vi "control_enabled_state.vi"(8 "error in (no error)":errorcluster, 10 "enabled":bool, 11 "control in":refnum<vi>) -> (0 "error out":errorcluster, 1 "disabled":bool, 2 "enabled":bool, 3 "control out":refnum<vi>)   [LabVIEW 2013, in "dsdll.lvlib"]
doc: "Enables or disables and grays references control."
uses:
  dsdll.lvlib
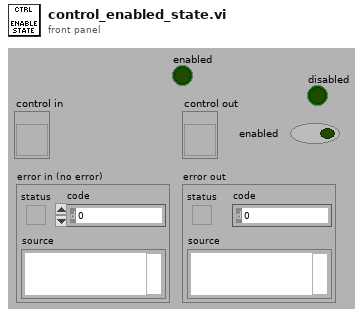
[diagram p1: front panel]
types:
  T1 = enum8{"Enabled", "Disabled", "Disabled and Grayed Out"}
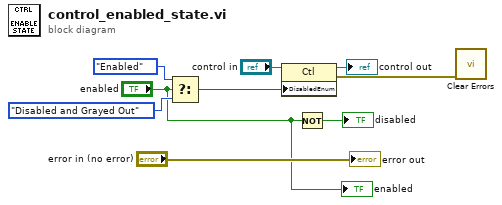
[diagram p0: block diagram]
diagram:
  n1 = Select(t=T1."Enabled" ("Disabled"), s="enabled", f=T1."Disabled and Grayed Out" ("Disabled")) -> (s? t:f=w8:T1)
  n2 = property class="Ctl"(reference="control in", "DisabledEnum"=w8) -> (reference out=→"control out":refnum<vi>, error out=w3:errorcluster)  [unwired: 1 in]
  n3 = Not(x="enabled") -> (.not. x?=→"disabled":bool)
  n4 = call <vilib>:"Clear Errors.vi"("error in (no error)"=w3) -> ()  [unwired: 6 in, 1 out]
  "error out" <- "error in (no error)"
  "enabled" <- "enabled"
